vi "Read (Single Point).vi"(0 "VISA resource name":refnum<visa-resource-name>, 5 "Timeout (10000 ms)":i32=10000 format="%#.6g", 11 "error in (no error)":errorcluster) -> (3 "Voltage":sgl, 4 "VISA resource name out":refnum<visa-resource-name>, 6 "Current":sgl, 8 "Resistance":sgl, 10 "Timestamp":sgl, 14 "Status":sgl, 15 "error out":errorcluster)   [LabVIEW 2009, in "Keithley 24XX.lvlib"]
doc: "Reads and returns a single measurement from the instrument.\n\n<B>Note:</B> Using this VI will overwrite all triggering settings with settings for a single point taken immediately. For control over the trigger, use the Low Level API."
uses:
  <instrlib>/Keithley 24XX/Keithley 24XX.lvlib
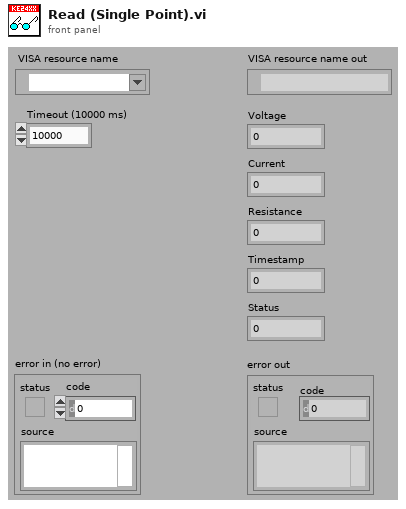
[diagram p1: front panel]
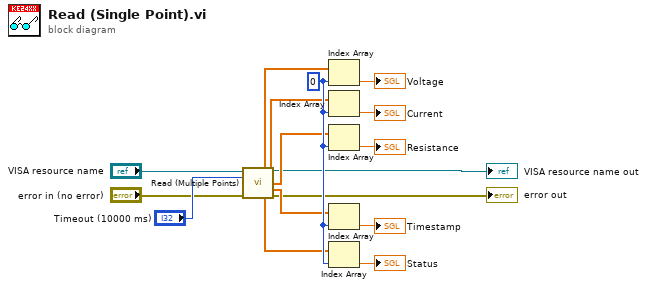
[diagram p0: block diagram]
diagram:
  w16 = 0 ("index")
  n1 = call "Read (Multiple Points).vi"("VISA resource name"="VISA resource name", "Timeout (10000 ms)"="Timeout (10000 ms)", "error in (no error)"="error in (no error)") -> ("Voltage"=w15:sgl[], "VISA resource name out"=→"VISA resource name out":refnum<visa-resource-name>, "Current"=w14:sgl[], "Resistance"=w13:sgl[], "Timestamp"=w12:sgl[], "Status"=w11:sgl[], "error out"=→"error out":errorcluster)  [unwired: 6 in]
  n2 = Index Array(array=w15, index=w16) -> (element=→"Voltage":sgl)
  n3 = Index Array(array=w14, index=w16) -> (element=→"Current":sgl)
  n4 = Index Array(array=w13, index=w16) -> (element=→"Resistance":sgl)
  n5 = Index Array(array=w12, index=w16) -> (element=→"Timestamp":sgl)
  n6 = Index Array(array=w11, index=w16) -> (element=→"Status":sgl)
